vi "ConvertRGBtoHSL.vi"() -> ()   [LabVIEW 2021]
panel:
  in  "B":u8
  in  "G":u8
  in  "R":u8
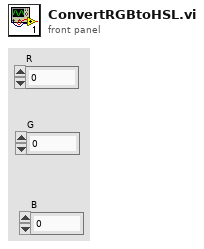
[diagram p1: front panel]
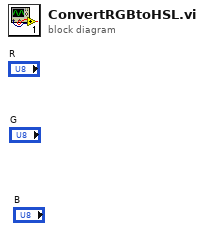
[diagram p0: block diagram]
diagram:
